vi "UsrProfiles-Prevent user name dupl.vi"(9 "User name ref":refnum<vi>, 11 "OK button ref":refnum<vi>) -> ()   [LabVIEW 2020]
panel:
  out "User Name":string
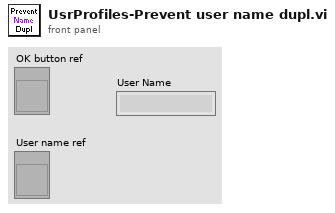
[diagram p1: front panel]
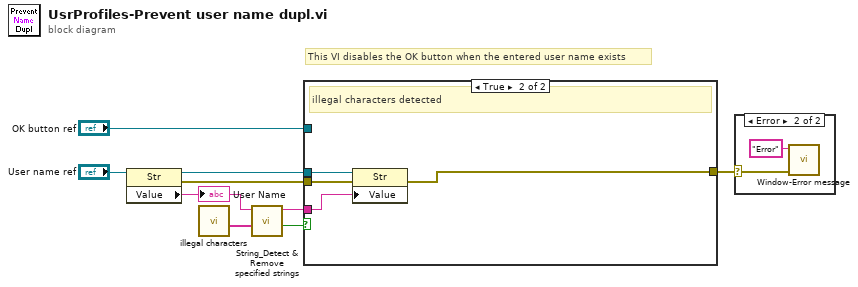
[diagram p0: block diagram]
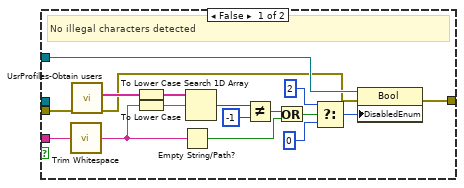
[diagram p3: hidden frame]
diagram:
  # "This VI disables the OK button when the entered user name exists"
  n1 = property class="Str"(reference="User name ref") -> (reference out=w2:refnum<vi>, error out=w3:errorcluster, "Value"=w4:string)  [unwired: 1 in]
  "User Name" <- w4
  n2 = call "illegal characters.vi"() -> ("Array of illegal characters"=w8:string[])  [unwired: 11 in]
  n3 = call <userlib>:"String_Detect & Remove specified strings.vi"("Array of illegal characters or whole words"=w8, "Input string"=w4) -> ("Illegal string detected"=w7:bool, "String with illegal elements removed"=w6:string)  [unwired: 8 in]
  n4 = case shown="True" w7 {
    tunnel: "OK button ref" -> [w18 _]
    tunnel: w6 -> [w13 w29]
    tunnel: w3 -> [w12 w28]
    tunnel: [w10 w27] -> w1
    tunnel: w2 -> [_ w30]
    frame False {
      # "No illegal characters detected"
      n5 = call <vilib>:"Trim Whitespace.vi"("string"=w13) -> ("trimmed string"=w17:string)  [unwired: 1 in]
      n6 = call "UsrProfiles-Obtain users.vi"("error in"=w12) -> ("error out"=w11:errorcluster, "User names"=w15:string[])  [unwired: 9 in]
      n7 = To Lower Case(string=w15) -> (all lower case string=w14:string[])
      n8 = To Lower Case(string=w17) -> (all lower case string=w16:string)
      n9 = Empty String/Path?(string/path=w17) -> (empty?=w22:bool)
      n10 = Search 1D Array(1D array=w14, element=w16) -> (index of element=w19:i32)  [unwired: 1 in]
      n11 = Not Equal?(x=w19, y=-1) -> (x != y?=w21:bool)
      n12 = Or(x=w21, y=w22) -> (x .or. y?=w23:bool)
      n13 = Select(t=2, s=w23, f=0) -> (s? t:f=w24:i32)
      n14 = property on="Property Node" class="Bool"(reference=w18, error in=w11, "DisabledEnum"=w24) -> (error out=w10:errorcluster)  [unwired: 1 out]
    }
    frame True {
      # "illegal characters detected"
      n15 = property class="Str"(reference=w30, error in=w28, "Value"=w29) -> (error out=w27:errorcluster)  [unwired: 1 out]
    }
  }
  n16 = case shown="Error" w1 {
    selector: w1 -> [_ w32]
    frame No Error {
    }
    frame Error {
      n17 = call "Window-Error message.vi"("error in (no error)"=w32, "Message"="Error") -> ()  [unwired: 9 in, 1 out]
    }
  }
